vi "Initialize.vi"(8 "Error In":errorcluster, 9 "Tolerance (m)":dbl, 10 "Round side?":enum16{"Starboard", "Port"}(ring), 11 "Buoy to Round":T1 {"North" format="%#_10f"; "East" format="%#_8f"}) -> (0 "Error Out":errorcluster, 3 "RoundBuoys out":refnum<class "RoundBuoy.lvclass">)   [LabVIEW 2011, in "RoundBuoy.lvclass"]
uses:
  RoundBuoy.lvclass
  2 Typedefs/UTM Location.ctl
  RoundBuoy.lvclass/RoundBuoy.ctl
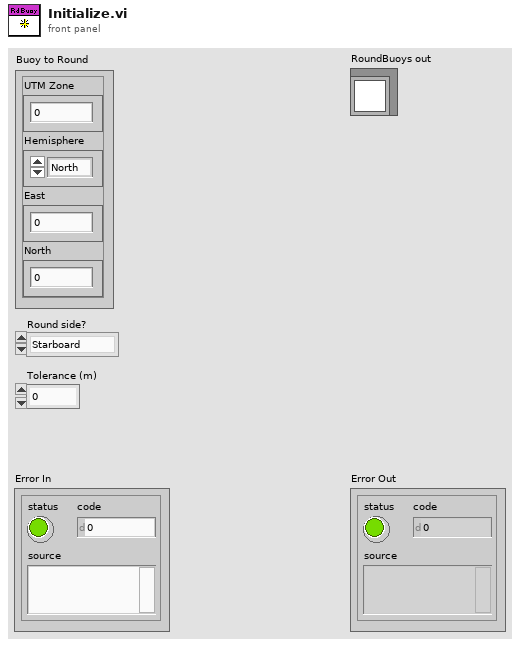
[diagram p1: front panel]
types:
  T1 = typedef "UTM Location.ctl" = cluster{"UTM Zone":dbl, "Hemisphere":enum16{"North", "South"}, "East":dbl, "North":dbl}
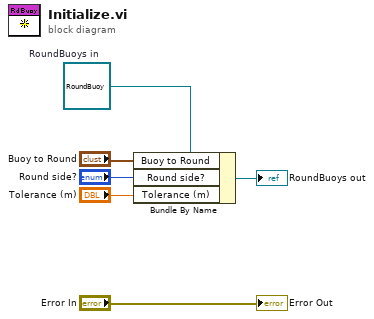
[diagram p0: block diagram]
diagram:
  w6 = refnum<class "RoundBuoy.lvclass"> refnum  # RoundBuoys in
  n1 = Bundle By Name(cluster=w6, "Buoy to Round"="Buoy to Round", "Round side?"="Round side?", "Tolerance (m)"="Tolerance (m)") -> (→"RoundBuoys out":refnum<class "RoundBuoy.lvclass">)
  "Error Out" <- "Error In"
